vi "Filter Event Data.vi"(8 "error in (no error)":errorcluster, 10 "EventFilter Reference":T1, 11 "ControlKeyDownMsg In":refnum<class "ControlKeyDownMsg.lvclass">) -> (0 "error out":errorcluster, 2 "Discard?":bool, 3 "ControlKeyDownMsg Out":refnum<class "ControlKeyDownMsg.lvclass">)   [LabVIEW 2019, in "ActorEvents.lvlib" / "ControlKeyDownMsg.lvclass"]
uses:
  <vilib>/gpm_packages/@cs/mva-viewable/Source/ActorEvents/IEventAggregator Messages/ControlKeyDownMsg/ControlKeyDownMsg.lvclass
  <vilib>/gpm_packages/@cs/mva-viewable/Source/ActorEvents/IEventFilter/EventFilter Reference.ctl
  <vilib>/gpm_packages/@cs/mva-viewable/Source/ActorEvents/IEventFilter/IEventFilter.lvclass
  <vilib>/gpm_packages/@cs/mva-viewable/Source/ActorEvents/IEventAggregator Messages/ControlKeyDownMsg/ControlKeyDownMsg.lvclass/ControlKeyDownMsg.ctl
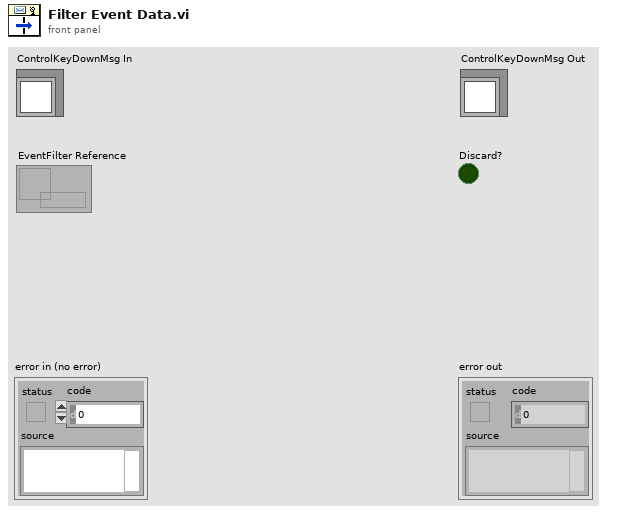
[diagram p1: front panel]
types:
  T1 = typedef "ActorEvents.lvlib/IEventFilter.lvclass/EventFilter Reference.ctl" = refnum<data-value>
  T2 = typedef "eventvkey.ctl" = enum16{"ASCII", "Enter", "Return", "Shift", "Ctrl", "Alt", "Cmd", "Opt", "Caps", "NumLock", "Clear", "Break", "Up", "Down", "Left", "Right", "Insert", "Delete", "Home", "End", "PageUp", "PageDown", "Escape", "Help", "Pause", "ScrollLock", "F1", "F2", "F3", "F4", "F5", "F6", "F7", "F8", "F9", "F10", "F11", "F12", "F13", "F14", "F15", "F16", "F17", "F18", "F19", "F20", "F21", "F22", "F23", "F24", "Play", "VolumeUp", "VolumeDown", "Mute", "Two Byte Char"}
  T3 = cluster{"Char":i16, "VKey":T2, "Mods":cluster{"Num Pad":bool, "Menu Key":bool}, "PlatMods":cluster{"Shift":bool, "Ctrl":bool, "Alt":bool, "Cmd":bool, "Opt":bool}, "FocusObj":refnum<vi>}
  T4 = cluster{"Shift":bool, "Ctrl":bool, "Alt":bool, "Cmd":bool, "Opt":bool}
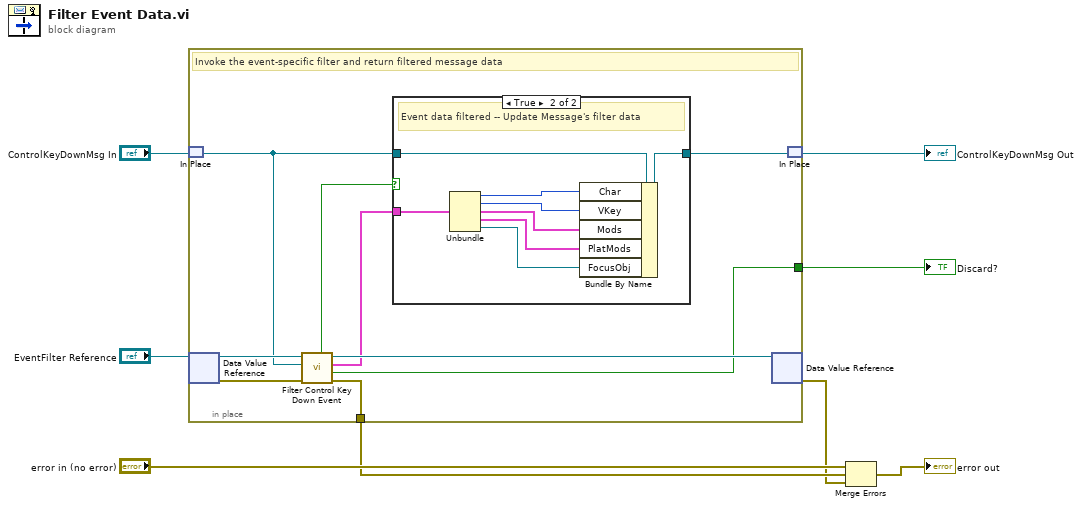
[diagram p0: block diagram]
diagram:
  n1 = in-place {
    in-place-border: [w13] -> w5
    in-place-border: [w14] -> w3
    # "Invoke the event-specific filter and return filtered message data"
    n2 = in-place-match #1("ControlKeyDownMsg In") -> (w11:refnum<class "ControlKeyDownMsg.lvclass">)
    n3 = in-place-dvr #2("EventFilter Reference") -> (w17:refnum<class "IEventFilter.lvclass">, w15:errorcluster)
    n4 = call-dynamic "Filter Control Key Down Event.vi"("error in (no error)"=w15, "ControlKeyDownMsg"=w11, "IEventFilter in"=w17) -> ("error out"=w13:errorcluster, "Discard?"=w14:bool, "Filtered Event Data"=w12:T3, "IEventFilter out"=w16:refnum<class "IEventFilter.lvclass">, "Data Filtered?"=w9:bool)  [unwired: 4 in]
    n5 = case shown="True" w9 {
      tunnel: w12 -> [_ w26]
      tunnel: w11 -> [w18 w20]
      tunnel: [w18 w19] -> w10
      frame False {
        # "No data filtered"
      }
      frame True {
        # "Event data filtered -- Update Message's filter data"
        n6 = Unbundle(w26) -> ("Char"=w25:i16, "VKey"=w24:T2, "Mods"=w23:cluster{"Num Pad":bool, "Menu Key":bool}, "PlatMods"=w22:T4, "FocusObj"=w21:refnum<vi>)
        n7 = Bundle By Name(cluster=w20, "Char"=w25, "VKey"=w24, "Mods"=w23, "PlatMods"=w22, "FocusObj"=w21) -> (w19:refnum<class "ControlKeyDownMsg.lvclass">)
      }
    }
    n8 = in-place-dvr #2(w16) -> (w4:errorcluster)  [unwired: 1 out]
    n9 = in-place-match #1(w10) -> (→"ControlKeyDownMsg Out":refnum<class "ControlKeyDownMsg.lvclass">)
  }
  "Discard?" <- w3
  n10 = Merge Errors("error in (no error)", w5, w4) -> (→"error out":errorcluster)
